vi "Main.vi"() -> ()   [LabVIEW 2021]
panel:
  in  "String":string
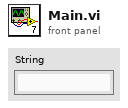
[diagram p1: front panel]
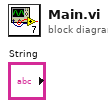
[diagram p0: block diagram]
diagram:
